vi "Configure Instrument.vi"(8 "error in (no error)":errorcluster, 11 "Example Instrument in":refnum<class "Example Instrument.lvclass">) -> (0 "error out":errorcluster, 3 "Example Instrument out":refnum<class "Example Instrument.lvclass">)   [LabVIEW 2016, in "Example Instrument.lvclass"]
uses:
  Example Instrument.lvclass
  Example Instrument.lvclass/Example Instrument.ctl
  <userlib>/LevyLab/Levylab Instruments/SMOs/Instrument/Instrument.lvclass
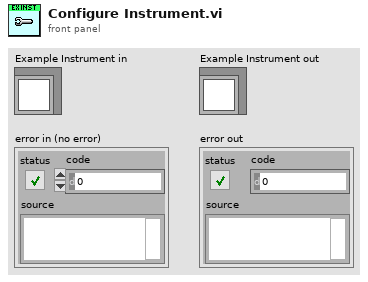
[diagram p1: front panel]
types:
  T1 = typedef "Example Instrument.lvclass/Configuration--Cluster.ctl" = cluster{"Example Setting 1":dbl, "Example Setting 2":dbl, "Example Setting 3":string}
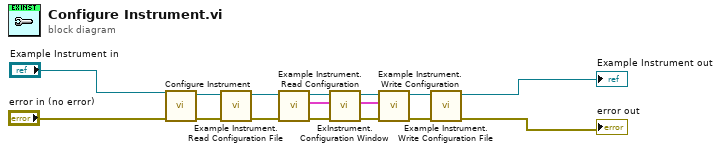
[diagram p0: block diagram]
diagram:
  n1 = call-parent "Configure Instrument.vi"("error in (no error)"="error in (no error)", "Instrument in"="Example Instrument in") -> ("error out"=w11:errorcluster, "Instrument out"=w13:refnum<class "Example Instrument.lvclass">)  [unwired: 8 in]
  n2 = call "Example Instrument.Read Configuration File.vi"("error in (no error)"=w11, "Example Instrument in"=w13) -> ("error out"=w10:errorcluster, "Example Instrument out"=w9:refnum<class "Example Instrument.lvclass">)  [unwired: 8 in]
  n3 = call "Example Instrument. Read Configuration.vi"("error in (no error)"=w10, "Example Instrument in"=w9) -> ("error out"=w7:errorcluster, "Ex Configuration"=w2:T1, "Example Instrument out"=w8:refnum<class "Example Instrument.lvclass">)  [unwired: 7 in]
  n4 = call-dynamic "ExInstrument.Configuration Window.vi"("error in (no error)"=w7, "Ex Configuration"=w2, "Example Instrument in"=w8) -> ("error out"=w6:errorcluster, "output cluster"=w1:T1, "Example Instrument out"=w5:refnum<class "Example Instrument.lvclass">)  [unwired: 6 in]
  n5 = call "Example Instrument. Write Configuration.vi"("error in (no error)"=w6, "Configuration"=w1, "Example Instrument in"=w5) -> ("error out"=w3:errorcluster, "Example Instrument out"=w4:refnum<class "Example Instrument.lvclass">)  [unwired: 7 in]
  n6 = call "Example Instrument.Write Configuration File.vi"("error in (no error)"=w3, "Example Instrument in"=w4) -> ("error out"=→"error out":errorcluster, "Example Instrument out"=→"Example Instrument out":refnum<class "Example Instrument.lvclass">)  [unwired: 8 in]
